vi "Set received proceed.vi"(8 "error in (no error)":errorcluster, 9 "from camera?":bool, 10 "from stage?":bool, 11 "Autofocus in":refnum<class "Autofocus.lvclass">) -> (0 "error out":errorcluster, 3 "Autofocus out":refnum<class "Autofocus.lvclass">)   [LabVIEW 2012, in "Autofocus.lvclass"]
uses:
  Autofocus.lvclass
  Autofocus.lvclass/Autofocus.ctl
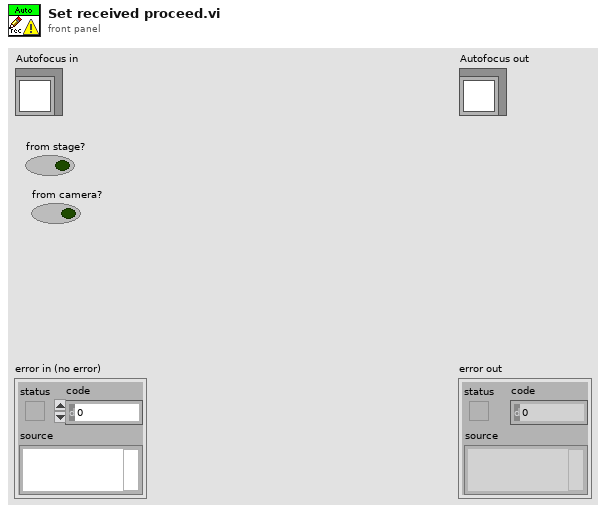
[diagram p1: front panel]
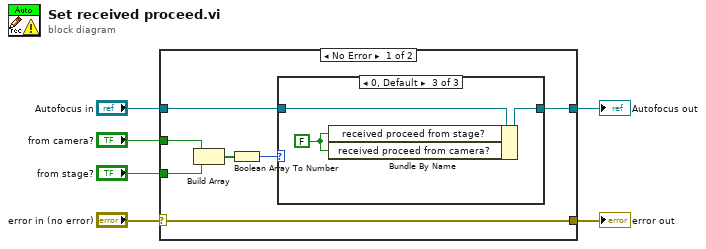
[diagram p0: block diagram]
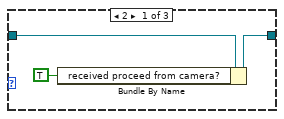
[diagram p2: hidden frame]
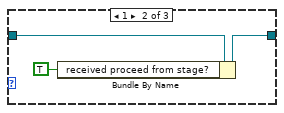
[diagram p3: hidden frame]
diagram:
  n1 = case shown="No Error" "error in (no error)" {
    selector: "error in (no error)" -> [w13 w24]
    tunnel: [w13 w24] -> w5
    tunnel: [w11 w23] -> w3
    tunnel: "Autofocus in" -> [w12 w23]
    tunnel: "from stage?" -> [w10 _]
    tunnel: "from camera?" -> [w9 _]
    frame No Error {
      n2 = Build Array(w9, w10) -> (w8:bool[])
      n3 = Boolean Array To Number(Boolean array=w8) -> (number=w7:u32)
      n4 = case shown="0, Default" w7 {
        tunnel: w12 -> [w16 w19 w22]
        tunnel: [w15 w18 w21] -> w11
        frame 2 {
          n5 = Bundle By Name(cluster=w16, "received proceed from camera?"=TRUE ("Runtime cluster.Checkpoint .received proceed from camera?")) -> (w15:refnum<class "Autofocus.lvclass">)
        }
        frame 1 {
          n6 = Bundle By Name(cluster=w19, "received proceed from stage?"=TRUE ("Runtime cluster.Checkpoint .received proceed from stage?")) -> (w18:refnum<class "Autofocus.lvclass">)
        }
        frame 0, Default {
          w20 = FALSE ("Runtime cluster.Checkpoint .received proceed from stage?")
          n7 = Bundle By Name(cluster=w22, "received proceed from stage?"=w20, "received proceed from camera?"=w20) -> (w21:refnum<class "Autofocus.lvclass">)
        }
      }
    }
    frame Error {
    }
  }
  "error out" <- w5
  "Autofocus out" <- w3
